vi "VI Tree.vi"   [LabVIEW 2015, in "Tektronix TDS 200 1000 2000 Series.lvlib"]
doc: "This is the instrument driver for Tektronix TDS 200, 1000, and 2000 Series oscilliscopes. The VI Tree displays all the user-callable VIs of the instrument driver in an organized table."
uses:
  <instrlib>/Tektronix TDS 200 1000 2000 Series/Tektronix TDS 200 1000 2000 Series.lvlib
  <instrlib>/Tektronix TDS 200 1000 2000 Series/Public/Configure/Configure Trigger (Edge).vi
  <instrlib>/Tektronix TDS 200 1000 2000 Series/Public/Data/Read (Single Waveform).vi
panel:
  # "(C) 2009-2015 National Instruments.  ALL RIGHTS RESERVED."
  # "SEE DIAGRAM\nFOR VI TREE."
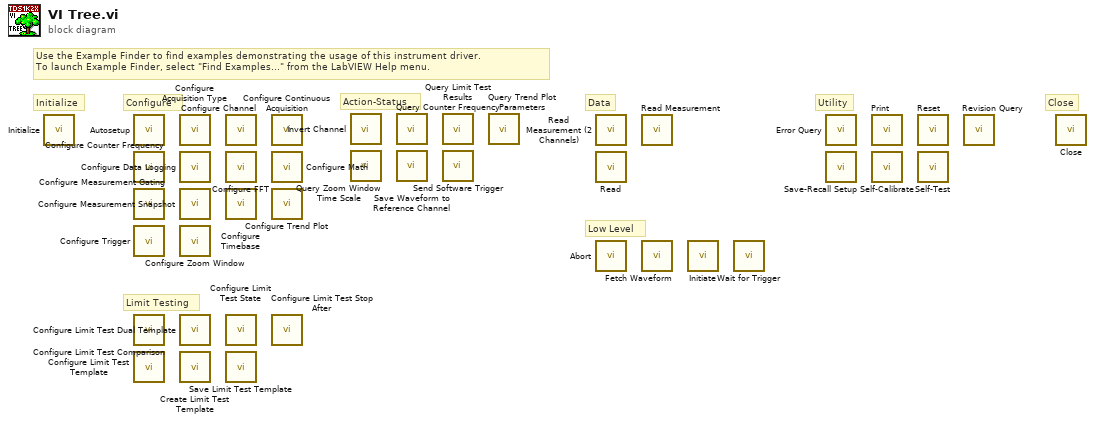
[diagram p0: block diagram]
diagram:
  # "Close"
  # "Utility"
  # "Low Level"
  # "Data"
  # "Limit Testing"
  # "Configure"
  # "Action-Status"
  # "Initialize"
  # "Use the Example Finder to find examples demonstrating the usage of this instrument driver.\nTo launch Example Finder, select \"Find Examples...\" from the LabVIEW Help menu."
  n1 = call <instrlib>:"Initialize.vi"() -> ()  [unwired: 10 in, 2 out]
  n2 = call <instrlib>:"Autosetup.vi"() -> ()  [unwired: 10 in, 2 out]
  n3 = call <instrlib>:"Configure Counter Frequency.vi"() -> ()  [unwired: 10 in, 2 out]
  n4 = call <instrlib>:"Configure Measurement Gating.vi"() -> ()  [unwired: 10 in, 2 out]
  n5 = call-poly <instrlib>:"Configure Trigger.vi"() -> ()  [unwired: 14 in, 2 out]
  n6 = call <instrlib>:"Configure Limit Test Comparison.vi"() -> ()  [unwired: 10 in, 2 out]
  n7 = call <instrlib>:"Configure Limit Test Template.vi"() -> ()  [unwired: 10 in, 2 out]
  n8 = call <instrlib>:"Configure Acquisition Type.vi"() -> ()  [unwired: 10 in, 2 out]
  n9 = call <instrlib>:"Configure Data Logging.vi"() -> ()  [unwired: 10 in, 2 out]
  n10 = call <instrlib>:"Configure Measurement Snapshot.vi"() -> ()  [unwired: 10 in, 2 out]
  n11 = call <instrlib>:"Configure Zoom Window.vi"() -> ()  [unwired: 10 in, 2 out]
  n12 = call <instrlib>:"Configure Limit Test Dual Template.vi"() -> ()  [unwired: 10 in, 2 out]
  n13 = call <instrlib>:"Create Limit Test Template.vi"() -> ()  [unwired: 10 in, 2 out]
  n14 = call <instrlib>:"Configure Channel.vi"() -> ()  [unwired: 14 in, 2 out]
  n15 = call <instrlib>:"Configure FFT.vi"() -> ()  [unwired: 10 in, 2 out]
  n16 = call <instrlib>:"Configure Timebase.vi"() -> ()  [unwired: 10 in, 2 out]
  n17 = call <instrlib>:"Configure Limit Test State.vi"() -> ()  [unwired: 10 in, 2 out]
  n18 = call <instrlib>:"Save Limit Test Template.vi"() -> ()  [unwired: 10 in, 2 out]
  n19 = call <instrlib>:"Configure Continuous Acquisition.vi"() -> ()  [unwired: 10 in, 2 out]
  n20 = call <instrlib>:"Configure Math.vi"() -> ()  [unwired: 10 in, 2 out]
  n21 = call <instrlib>:"Configure Trend Plot.vi"() -> ()  [unwired: 10 in, 2 out]
  n22 = call <instrlib>:"Configure Limit Test Stop After.vi"() -> ()  [unwired: 10 in, 2 out]
  n23 = call <instrlib>:"Invert Channel.vi"() -> ()  [unwired: 10 in, 2 out]
  n24 = call <instrlib>:"Query Zoom Window Time Scale.vi"() -> ()  [unwired: 9 in, 3 out]
  n25 = call <instrlib>:"Query Counter Frequency.vi"() -> ()  [unwired: 9 in, 3 out]
  n26 = call <instrlib>:"Save Waveform to Reference Channel.vi"() -> ()  [unwired: 10 in, 2 out]
  n27 = call <instrlib>:"Query Limit Test Results.vi"() -> ()  [unwired: 7 in, 5 out]
  n28 = call <instrlib>:"Send Software Trigger.vi"() -> ()  [unwired: 10 in, 2 out]
  n29 = call <instrlib>:"Query Trend Plot Parameters.vi"() -> ()  [unwired: 6 in, 10 out]
  n30 = call <instrlib>:"Read Measurement (2 Channels).vi"() -> ()  [unwired: 8 in, 4 out]
  n31 = call-poly <instrlib>:"Read.vi"() -> ()  [unwired: 9 in, 3 out]
  n32 = call <instrlib>:"Abort.vi"() -> ()  [unwired: 10 in, 2 out]
  n33 = call <instrlib>:"Read Measurement.vi"() -> ()  [unwired: 8 in, 4 out]
  n34 = call <instrlib>:"Fetch Waveform.vi"() -> ()  [unwired: 9 in, 3 out]
  n35 = call <instrlib>:"Initiate.vi"() -> ()  [unwired: 10 in, 2 out]
  n36 = call <instrlib>:"Wait for Trigger.vi"() -> ()  [unwired: 10 in, 2 out]
  n37 = call <instrlib>:"Error Query.vi"() -> ()  [unwired: 8 in, 4 out]
  n38 = call <instrlib>:"Save-Recall Setup.vi"() -> ()  [unwired: 10 in, 2 out]
  n39 = call <instrlib>:"Print.vi"() -> ()  [unwired: 10 in, 2 out]
  n40 = call <instrlib>:"Self-Calibrate.vi"() -> ()  [unwired: 9 in, 3 out]
  n41 = call <instrlib>:"Reset.vi"() -> ()  [unwired: 10 in, 2 out]
  n42 = call <instrlib>:"Self-Test.vi"() -> ()  [unwired: 8 in, 4 out]
  n43 = call <instrlib>:"Revision Query.vi"() -> ()  [unwired: 8 in, 4 out]
  n44 = call <instrlib>:"Close.vi"() -> ()  [unwired: 11 in, 1 out]
